vi "GetProgramTime.vi"(8 "error in":errorcluster, 11 "VISA resource name":refnum<visa-resource-name>) -> (0 "error out":errorcluster, 2 "Program time":string, 3 "VISA resource name out":refnum<visa-resource-name>)   [LabVIEW 2023, in "Thermotron 8800.lvlib"]
doc: "PTIM\nCommand name: Send program time\nCommand type: Program status\nDescription: Queries the 8800 for the total estimated time for the current program.\nSyntax: PTIM?\nData type: String\nQuery example: PTIM?\n8800 response: 48:30:10 (The current program is 48 hours, 30 minutes, 10 seconds long.)"
uses:
  Thermotron 8800.lvlib
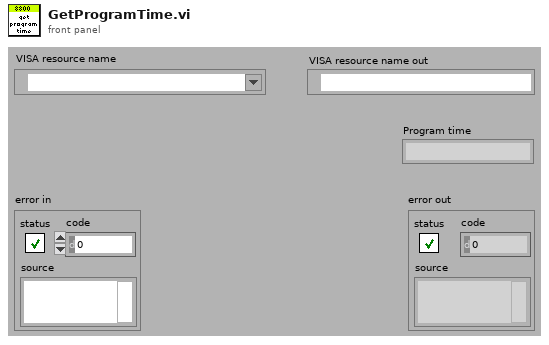
[diagram p1: front panel]
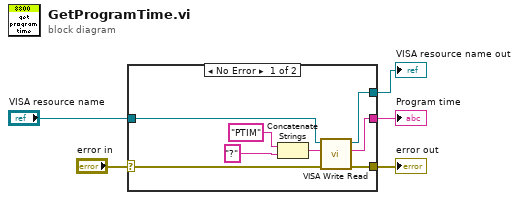
[diagram p0: block diagram]
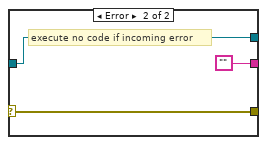
[diagram p2: hidden frame]
diagram:
  n1 = case shown="No Error" "error in" {
    selector: "error in" -> [w11 w15]
    tunnel: [w8 w15] -> w4
    tunnel: [w9 w16] -> w3
    tunnel: "VISA resource name" -> [w10 w16]
    tunnel: [w7 ""] -> w1
    frame No Error {
      n2 = Concatenate Strings("PTIM" ("8800 Command"), "?" ("8800 Command")) -> (w13:string)
      n3 = call "VISA Write Read.vi"("error in (no error)"=w11, "8800 Command"=w13, "VISA Refnum in"=w10) -> ("error out"=w8:errorcluster, "read buffer"=w7:string, "VISA Refnum out"=w9:refnum<visa-resource-name>)  [unwired: 6 in]
    }
    frame Error {
      # "execute no code if incoming error"
    }
  }
  "VISA resource name out" <- w3
  "error out" <- w4
  "Program time" <- w1
